vi "GetSystemsStatus.vi"() -> (0 "All systems offline?":bool, 1 "All systems online?":bool, 2 "Thread States":T2, 3 "Systems Online":T3)   [LabVIEW 2015]
uses:
  SystemUtil/ThreadStates.ctl
  Wavelength/GSP_Wavelength_Global.vi
  TCS_Link/TCSLINK_global.vi
  Grating_Translation/GSP_GT_Global.vi
  Slit/GSP_SLIT_Global.vi
  Primary Filter/GSP_F1_Global.vi
  Secondary Filter/GSP_F2_Global.vi
  Coll_Focus/GSP_COLL_Global.vi
  Cam_Focus/GSP_CF_Global.vi
  Log/GSP_Logger_Global.vi
  SIcamera_Control/Apogee_Global.vi
  TCPServer/TCPServer_Global.vi
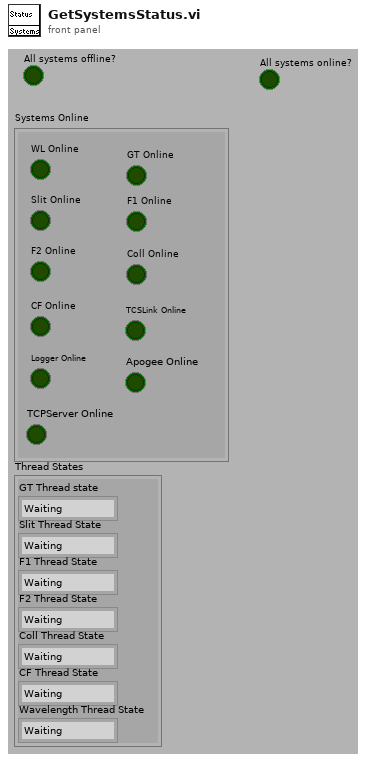
[diagram p1: front panel]
types:
  T1 = typedef "ThreadStates.ctl" = enum16{"Waiting", "Scripting", "Uninitialized", "Error"}
  T2 = cluster{"GT Thread state":T1, "Slit Thread State":T1, "F1 Thread State":T1, "F2 Thread State":T1, "Coll Thread State":T1, "CF Thread State":T1, "Wavelength Thread State":T1}
  T3 = cluster{"WL Online":bool, "GT Online":bool, "Slit Online":bool, "F1 Online":bool, "F2 Online":bool, "Coll Online":bool, "CF Online":bool, "TCSLink Online":bool, "Logger Online":bool, "Apogee Online":bool, "TCPServer Online":bool}
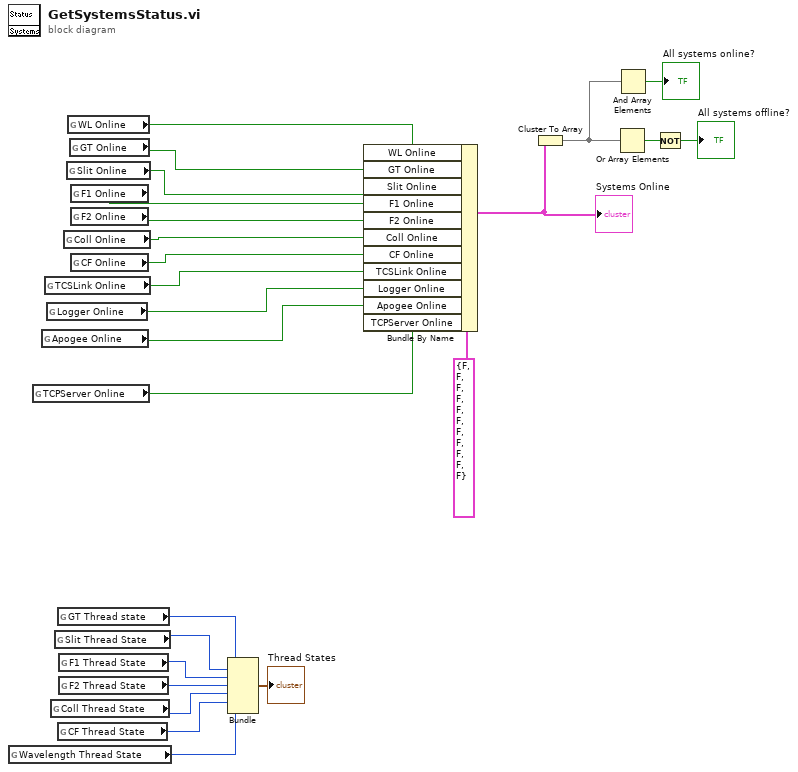
[diagram p0: block diagram]
diagram:
  n1 = global read "GSP_Wavelength_Global.vi" "Wavelength Thread State"() -> (w2:T1)
  n2 = global read "TCPServer_Global.vi" "TCPServer Online"() -> (w9:bool)
  n3 = global read "Apogee_Global.vi" "Apogee Online"() -> (w10:bool)
  n4 = global read "TCSLINK_global.vi" "TCSLink Online"() -> (w18:bool)
  n5 = global read "GSP_Logger_Global.vi" "Logger Online"() -> (w15:bool)
  n6 = global read "GSP_COLL_Global.vi" "Coll Thread State"() -> (w4:T1)
  n7 = global read "GSP_SLIT_Global.vi" "Slit Thread State"() -> (w7:T1)
  n8 = global read "GSP_GT_Global.vi" "GT Thread state"() -> (w8:T1)
  n9 = global read "GSP_CF_Global.vi" "CF Thread State"() -> (w3:T1)
  n10 = global read "GSP_F1_Global.vi" "F1 Thread State"() -> (w6:T1)
  n11 = global read "GSP_F2_Global.vi" "F2 Thread State"() -> (w5:T1)
  n12 = global read "GSP_COLL_Global.vi" "Coll Online"() -> (w20:bool)
  n13 = global read "GSP_SLIT_Global.vi" "Slit Online"() -> (w23:bool)
  n14 = global read "GSP_Wavelength_Global.vi" "WL Online"() -> (w21:bool)
  n15 = global read "GSP_GT_Global.vi" "GT Online"() -> (w22:bool)
  n16 = global read "GSP_F1_Global.vi" "F1 Online"() -> (w25:bool)
  n17 = global read "GSP_F2_Global.vi" "F2 Online"() -> (w24:bool)
  n18 = global read "GSP_CF_Global.vi" "CF Online"() -> (w19:bool)
  n19 = Bundle("GT Thread state"=w8, "Slit Thread State"=w7, "F1 Thread State"=w6, "F2 Thread State"=w5, "Coll Thread State"=w4, "CF Thread State"=w3, "Wavelength Thread State"=w2) -> (→"Thread States":T2)  [unwired: 1 in]
  n20 = Bundle By Name(cluster=T3 {"WL Online"=FALSE, "GT Online"=FALSE, "Slit Online"=FALSE, "F1 Online"=FALSE, "F2 Online"=FALSE, "Coll Online"=FALSE, "CF Online"=FALSE, "TCSLink Online"=FALSE, "Logger Online"=FALSE, "Apogee Online"=FALSE, "TCPServer Online"=FALSE} ("Systems Status"), "WL Online"=w21, "GT Online"=w22, "Slit Online"=w23, "F1 Online"=w25, "F2 Online"=w24, "Coll Online"=w20, "CF Online"=w19, "TCSLink Online"=w18, "Logger Online"=w15, "Apogee Online"=w10, "TCPServer Online"=w9) -> (w11:T3)
  "Systems Online" <- w11
  n21 = Cluster To Array(cluster=w11) -> (array=w14:bool[])
  n22 = Or Array Elements(Boolean array=w14) -> (logical OR=w17:bool)
  n23 = And Array Elements(Boolean array=w14) -> (logical AND=→"All systems online?":bool)
  n24 = Not(x=w17) -> (.not. x?=→"All systems offline?":bool)
